vi "New Server Test.vi"() -> ()   [LabVIEW 2019]
uses:
  <vilib>/Utility/file.llb/Write To Spreadsheet File (DBL).vi
panel:
  out "error out":errorcluster
  in  "Test Name":string="Test Name"
  in  "CA Number":string="CA Number"
  in  "Date":string="Date"
  in  "Filename":string="Transfer Test.csv"
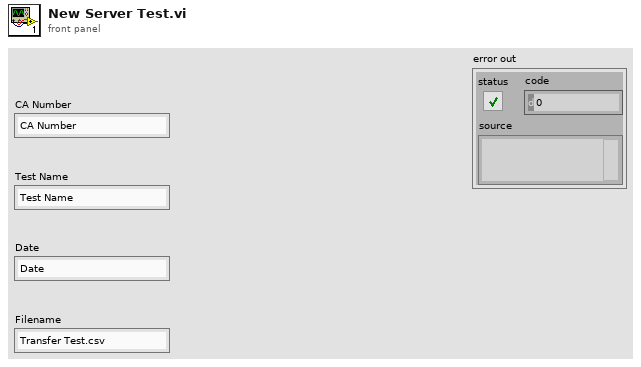
[diagram p1: front panel]
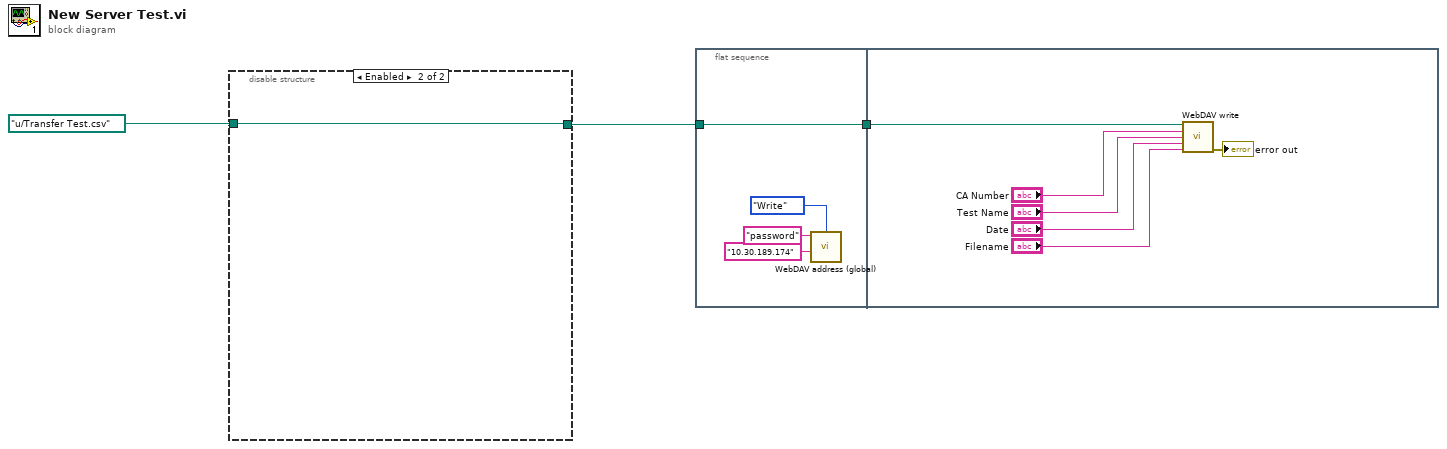
[diagram p0: block diagram]
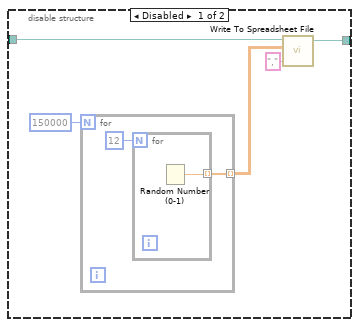
[diagram p2: hidden frame]
diagram:
  n1 = disable-structure shown="Enabled" {
    disable-tunnel: path "u:/Transfer Test.csv" -> [w8 w12]
    disable-tunnel: [w7 w12] -> w1
    frame Disabled {
      n2 = for {
        N: 150000 -> [_]
        tunnel: [w9] -> w5 mode=indexing
        n3 = for {
          N: 12 -> [_]
          tunnel: [w11] -> w9 mode=indexing
          n4 = Random Number (0-1)() -> (number: 0 to 1=w11:dbl)
        }
      }
      n5 = call-poly <vilib>:"Write To Spreadsheet File.vi"("delimiter (\\t)"="," ("delimiter (\\t)"), "2D data"=w5, "file path (dialog if empty)"=w8) -> ("new file path (Not A Path if cancelled)"=w7:path)  [unwired: 5 in]
    }
    frame Enabled {
    }
  }
  n6 = flat-sequence {
    tunnel: [w13] -> w2
    tunnel: w1 -> [w13]
    tunnel: w2 -> [w17]
    frame #0 {
      n7 = call "WebDAV address (global).vi"("Mode"=enum16{"Read", "Write"}."Write", "Network Drive Password"="password", "Network Drive IP"="10.30.189.174") -> ()  [unwired: 5 in, 2 out]
    }
    frame #1 {
      n8 = call "WebDAV write.vi"("RIO Filepath"=w17, "CA Number"="CA Number", "Test Name"="Test Name", "Date"="Date", "Filename"="Filename") -> ("error out"=→"error out":errorcluster)  [unwired: 10 in]
    }
  }
